vi "Find Implemented Msgs.vi"(10 "Path":path) -> (2 "Implemented Msgs":T1)   [LabVIEW 2020, in "jettl.lvlib" / "Actor.lvlib"]
uses:
  Actor.lvlib
  Msg/Msg.lvclass
  Implemented Msgs.ctl
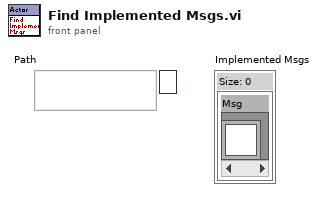
[diagram p1: front panel]
types:
  T1 = typedef "jettl.lvlib/Actor.lvlib/Implemented Msgs.ctl" = set{refnum<class "Msg.lvclass">}
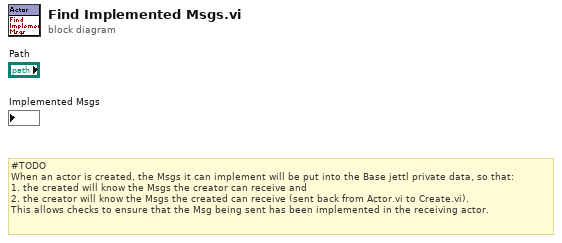
[diagram p0: block diagram]
diagram:
  # "#TODO\nWhen an actor is created, the Msgs it can implement will be put into the Base jettl private data, so that:\n1. the created will know the Msgs the creator can receive and\n2. the creator will know the Msgs the created can receive (sent back from Actor.vi to Create.vi).\nThis allows checks to ensure that the Msg being sent has been implemented in the receiving actor."
